vi "Handle Error.vi"(8 "error in (no error)":errorcluster, 11 "DAM0404D in":refnum<class "DAM0404D.lvclass">) -> (0 "error out":errorcluster, 2 "stop actor?":bool=TRUE, 3 "DAM0404D out":refnum<class "DAM0404D.lvclass">)   [LabVIEW 2016, in "DAM0404D.lvlib" / "DAM0404D.lvclass"]
doc: "(<B>Filename</B>: Actor Framework.lvlib:Actor.lvclass:Handle Error.vi)\n\nDefines how the actor handles an error that occurred while processing a message. By default, this method does nothing except stop the actor."
uses:
  DAM0404D.lvclass
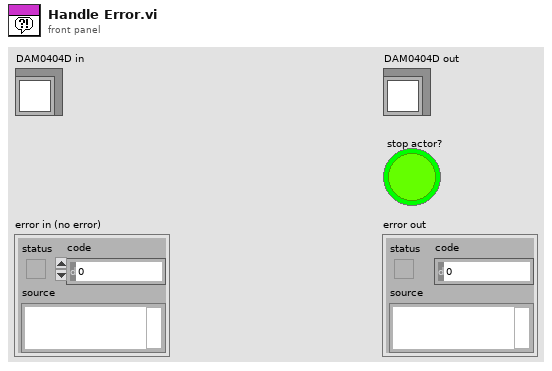
[diagram p1: front panel]
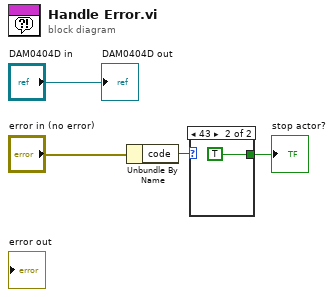
[diagram p0: block diagram]
diagram:
  n1 = Unbundle By Name("error in (no error)") -> ("code"=w3:i32)
  n2 = case shown="43" w3 {
    tunnel: [_ TRUE] -> w2
    frame 0, Default {
    }
    frame 43 {
    }
  }
  "stop actor?" <- w2
  "DAM0404D out" <- "DAM0404D in"
